vi "get SNR.vi"(8 "SNR threshold":dbl, 10 "Refnum in":T1, 11 "fifo ready":bool) -> (0 "packet valid now":bool, 1 "noise power":dbl, 2 "signal power":dbl, 3 "FPGA VI Reference Out":T1, 4 "packet valid":bool, 5 "SNR":dbl)   [LabVIEW 2020]
uses:
  Host/SubVIs/Streaming Xvcr FPGA Ref.ctl
  <vilib>/Utility/error.llb/Error Cluster From Error Code.vi
  <vilib>/rvi/errors/niLvFpgaAdjustHostInterfaceError.vi
  <vilib>/rvi/interface/nirviMethod/nirviMethod.xnode
  <vilib>/FPGAPlugInAG/Dynamic/niLvFpga_ReadFifo_Dynamic.vi
  <vilib>/rvi/errors/niLvFpgaMergeErrorWithErrorCode.vi
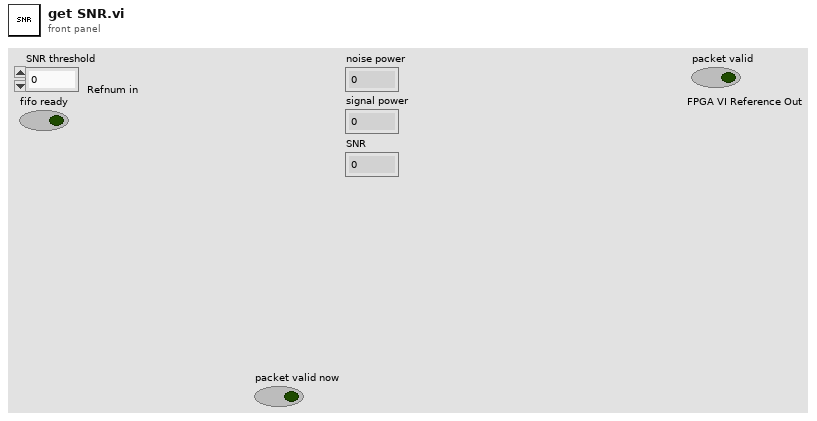
[diagram p1: front panel]
types:
  T1 = typedef "Streaming Xvcr FPGA Ref.ctl" = refnum<k20>
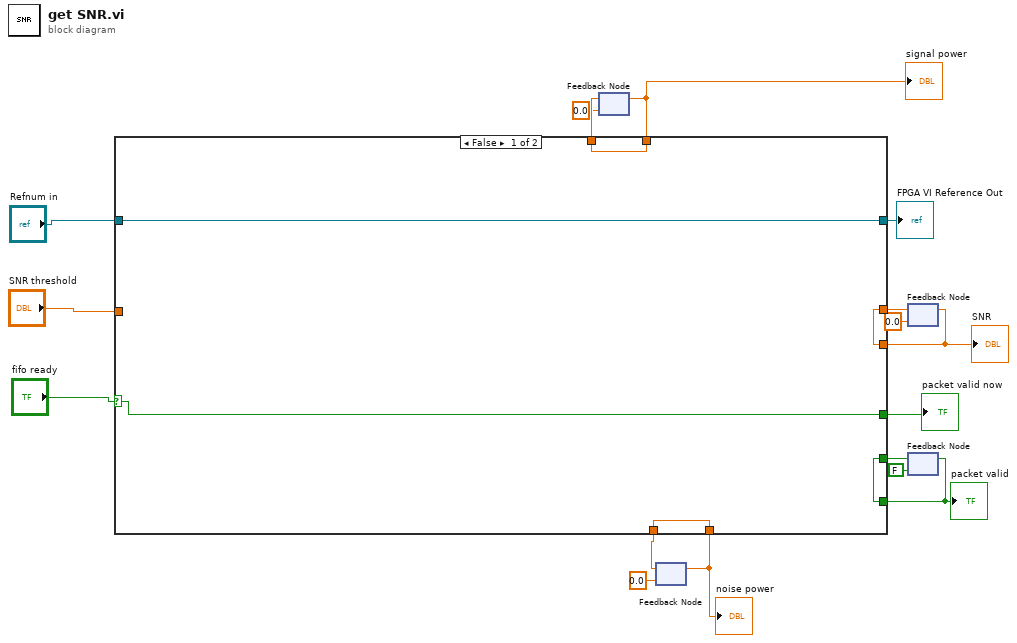
[diagram p0: block diagram]
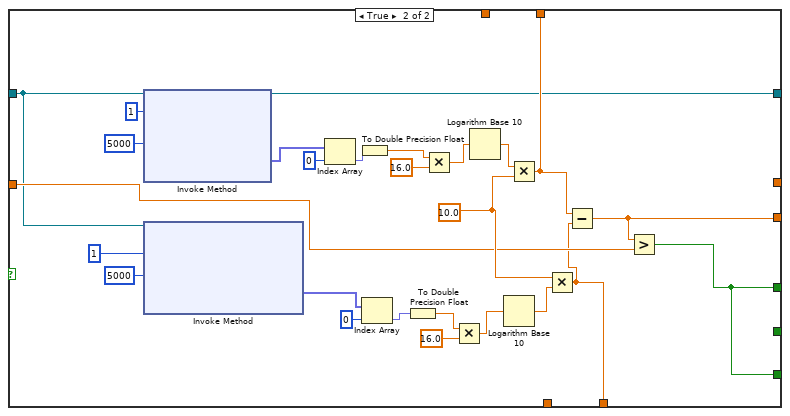
[diagram p2: hidden frame]
diagram:
  n1 = feedback #1(0.0) -> (w10:dbl)
  n2 = feedback #2(0.0) -> (w8:dbl)
  n3 = feedback #3(0.0) -> (w12:dbl)
  n4 = feedback #4(FALSE) -> (w2:bool)
  n5 = case shown="False" "fifo ready" {
    selector: "fifo ready" -> [w20 _]
    tunnel: "SNR threshold" -> [_ w30]
    tunnel: "Refnum in" -> [w18 w29]
    tunnel: [w20 w25] -> w15
    tunnel: [w21 w28] -> w13
    tunnel: [w23 w27] -> w11
    tunnel: [w22 w26] -> w9
    tunnel: w12 -> [w21 _]
    tunnel: w10 -> [w23 _]
    tunnel: w8 -> [w22 _]
    tunnel: [w19 w25] -> w4
    tunnel: w2 -> [w19 _]
    tunnel: [w18 w24] -> w1
    frame False {
    }
    frame True {
      w49 = 10.0 ("x")
      n6 = xnode "Invoke Method"("FPGA VI Reference In"=w29, "Number of Elements"=u32 1, "Timeout (ms)"=5000) -> ("FPGA VI Reference Out"=w24:T1, "Data"=w42:fxp<+,38,6>[])  [unwired: 1 in, 2 out]
      n7 = xnode "Invoke Method"("FPGA VI Reference In"=w29, "Number of Elements"=u32 1, "Timeout (ms)"=5000) -> ("Data"=w38:fxp<+,38,6>[])  [unwired: 1 in, 3 out]
      n8 = Index Array(array=w42, index=0) -> (element=w40:fxp<+,38,6>)
      n9 = To Double Precision Float(number=w40) -> (double precision float=w32:dbl)
      n10 = Index Array(array=w38, index=0) -> (element=w37:fxp<+,38,6>)
      n11 = To Double Precision Float(number=w37) -> (double precision float=w35:dbl)
      n12 = Multiply(x=w32, y=16.0) -> (x*y=w31:dbl)
      n13 = Multiply(x=w35, y=16.0) -> (x*y=w34:dbl)
      n14 = Logarithm Base 10(1:w31) -> (0:w47:dbl)
      n15 = Logarithm Base 10(1:w34) -> (0:w48:dbl)
      n16 = Multiply(x=w47, y=w49) -> (x*y=w27:dbl)
      n17 = Multiply(x=w49, y=w48) -> (x*y=w26:dbl)
      n18 = Subtract(x=w27, y=w26) -> (x-y=w28:dbl)
      n19 = Greater?(x=w28, y=w30) -> (0:w25:bool)
    }
  }
  "packet valid now" <- w15
  "signal power" <- w11
  "SNR" <- w13
  "noise power" <- w9
  "packet valid" <- w4
  "FPGA VI Reference Out" <- w1
  n20 = feedback-in #1(w11) -> ()
  n21 = feedback-in #2(w9) -> ()
  n22 = feedback-in #3(w13) -> ()
  n23 = feedback-in #4(w4) -> ()
